vi "Read all info -- subVI.vi"(8 "error in (no error)":errorcluster, 11 "VISA Refnum in":refnum<visa-resource-name>) -> (0 "error out":errorcluster, 1 "End-position?":bool, 2 "End-stops":cluster{"ES1":bool, "ES2":bool}, 3 "Position":i32, 5 "Home?":bool)   [LabVIEW 2020, in "Arduino stepper.lvlib"]
uses:
  Arduino stepper.lvlib
  <vilib>/Instr/_visa.llb/VISA Flush IO Buffer Mask.ctl
panel:
  out "read buffer":string
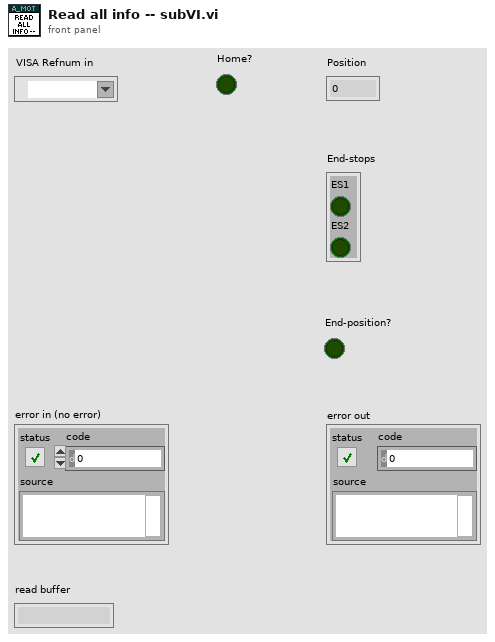
[diagram p1: front panel]
types:
  T1 = typedef "VISA Flush IO Buffer Mask.ctl" = u16
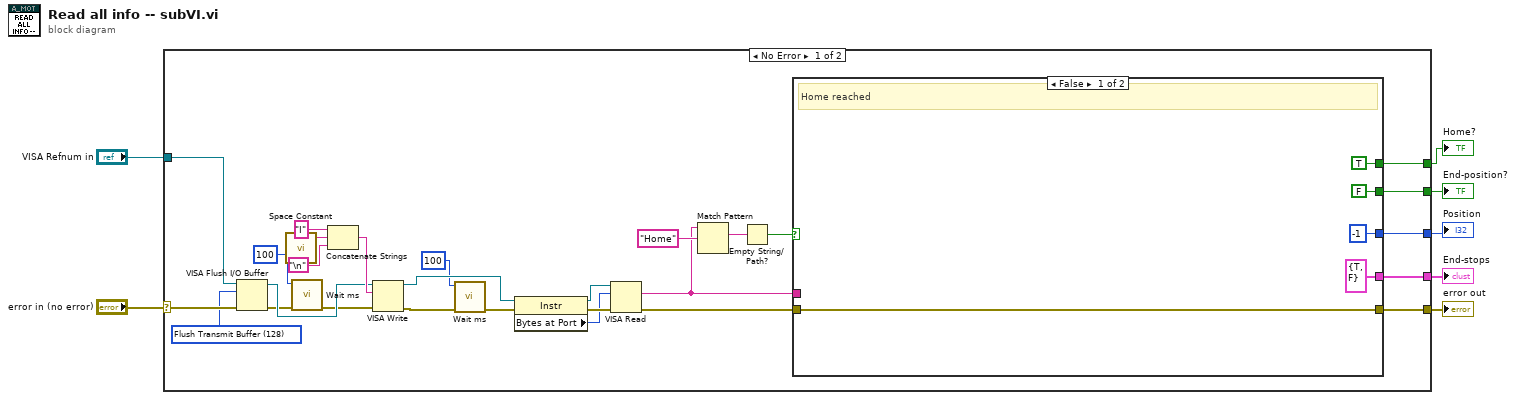
[diagram p0: block diagram]
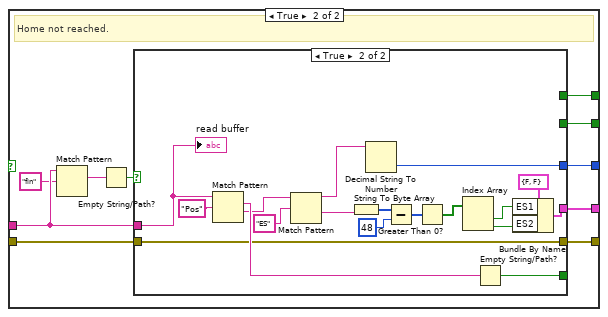
[diagram p2: hidden frame]
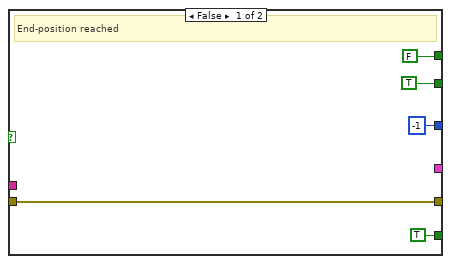
[diagram p3: hidden frame]
diagram:
  n1 = case shown="No Error" "error in (no error)" {
    selector: "error in (no error)" -> [w26 w74]
    tunnel: [w24 w74] -> w5
    tunnel: "VISA Refnum in" -> [w28 _]
    tunnel: [w21 _] -> w4
    tunnel: [w20 _] -> w3
    tunnel: [w13 _] -> w2
    tunnel: [w8 _] -> w1
    frame No Error {
      w23 = T1 128 items=["Flush Receive Buffer"=16, "Write Transmit Buffer to Device"=32, "Flush Receive Buffer (No I/O)"=64, "Flush Transmit Buffer"=128] ("Mask")
      n2 = VISA Flush I/O Buffer(VISA resource name=w28, mask (16)=w23, error in (no error)=w26) -> (VISA resource name out=w33:refnum<visa-resource-name>, error out=w27:errorcluster)
      n3 = call <vilib>:"Space Constant.vi"() -> ("String"=w22:string)
      n4 = call "Wait ms.vi"("error in (no error)"=w27, "milliseconds to wait"=u32 100) -> ("error out"=w32:errorcluster)  [unwired: 9 in]
      n5 = Concatenate Strings("I" ("string"), w22, "\n") -> (w34:string)
      n6 = VISA Write(VISA resource name=w33, write buffer=w34, error in (no error)=w32) -> (VISA resource name out=w25:refnum<visa-resource-name>, error out=w35:errorcluster)  [unwired: 1 out]
      n7 = call "Wait ms.vi"("error in (no error)"=w35, "milliseconds to wait"=u32 100) -> ("error out"=w18:errorcluster)  [unwired: 9 in]
      n8 = property class="Instr"(reference=w25, error in=w18) -> (reference out=w16:refnum<visa-resource-name>, error out=w17:errorcluster, "Bytes at Port"=w15:u32)
      n9 = VISA Read(VISA resource name=w16, byte count=w15, error in (no error)=w17) -> (read buffer=w9:string, error out=w14:errorcluster)  [unwired: 2 out]
      n10 = Match Pattern(string=w9, regular expression="Home") -> (match substring=w12:string)  [unwired: 1 in, 3 out]
      n11 = Empty String/Path?(string/path=w12) -> (empty?=w10:bool)
      n12 = case shown="False" w10 {
        tunnel: [w38 w50] -> w24
        tunnel: [-1 w49] -> w21
        tunnel: [cluster{"ES1":bool, "ES2":bool} {"ES1"=TRUE, "ES2"=FALSE} w48] -> w20
        tunnel: w9 -> [_ w47]
        tunnel: w14 -> [w38 w43]
        tunnel: [FALSE w42] -> w13
        tunnel: [TRUE w41] -> w8
        frame False {
          # "Home reached"
        }
        frame True {
          # "Home not reached."
          n13 = Match Pattern(string=w47, regular expression="fin") -> (match substring=w45:string)  [unwired: 1 in, 3 out]
          n14 = Empty String/Path?(string/path=w45) -> (empty?=w44:bool)
          n15 = case shown="True" w44 {
            tunnel: [TRUE w71] -> _
            tunnel: [-1 w67] -> w49
            tunnel: [_ w58] -> w48
            tunnel: w47 -> [_ w57]
            tunnel: w43 -> [w53 w56]
            tunnel: [w53 w56] -> w50
            tunnel: [TRUE _] -> w42
            tunnel: [FALSE _] -> w41
            frame False {
              # "End-position reached"
            }
            frame True {
              n16 = Match Pattern(string=w57, regular expression="Pos") -> (match substring=w72:string, after substring=w70:string)  [unwired: 1 in, 2 out]
              n17 = Match Pattern(string=w70, regular expression="ES") -> (before substring=w68:string, after substring=w59:string)  [unwired: 1 in, 2 out]
              n18 = String To Byte Array(string=w59) -> (unsigned byte array=w62:u8[])
              n19 = Decimal String To Number(string=w68) -> (number=w67:i32)  [unwired: 2 in, 1 out]
              n20 = Subtract(x=w62, y=u8 48) -> (x-y=w63:u8[])
              n21 = Greater Than 0?(x=w63) -> (x > 0?=w64:bool[])
              n22 = Index Array(array=w64) -> (element #1=w66:bool, element #2=w65:bool)  [unwired: 2 in]
              n23 = Empty String/Path?(string/path=w72) -> (empty?=w71:bool)
              n24 = Bundle By Name(cluster=cluster{"ES1":bool, "ES2":bool} {"ES1"=FALSE, "ES2"=FALSE}, "ES1"=w66, "ES2"=w65) -> (w58:cluster{"ES1":bool, "ES2":bool})
              "read buffer" <- w57
            }
          }
        }
      }
    }
    frame Error {
    }
  }
  "error out" <- w5
  "Position" <- w4
  "End-stops" <- w3
  "End-position?" <- w2
  "Home?" <- w1
